vi "GetSystemDirectory.vi"() -> ()   [LabVIEW 2011]
doc: "Uses an API call to retrieve the path to thesystem directory."
uses:
  kernel32.dll
panel:
  out "error out":errorcluster
  in  "error in (no error)":errorcluster
  out "System Directory Path":string
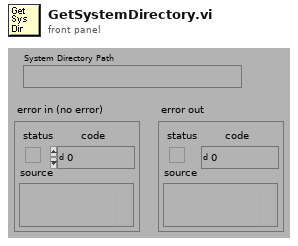
[diagram p1: front panel]
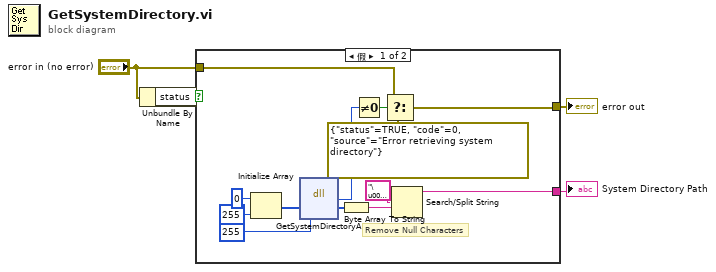
[diagram p0: block diagram]
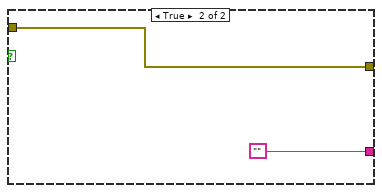
[diagram p2: hidden frame]
diagram:
  n1 = Unbundle By Name("error in (no error)") -> ("status"=w3:bool)
  n2 = case shown="假" w3 {
    tunnel: [w12 "" ("string")] -> w4
    tunnel: "error in (no error)" -> [w7 w19]
    tunnel: [w6 w19] -> w1
    frame False {
      # "Remove Null Characters"
      n3 = Initialize Array(u8 0, 255) -> (w15:u8[])
      n4 = dll-call lib="kernel32.dll" fn="GetSystemDirectoryA" label="Get System Directory"("lpBuffer"=w15, "nSize"=u32 255) -> (w9:u8, "lpBuffer"=w16:u8[])  [unwired: 4 in, 2 out]
      n5 = Byte Array To String(unsigned byte array=w16) -> (string=w14:string)
      n6 = Not Equal To 0?(x=w9) -> (x != 0?=w8:bool)
      n7 = Select(t=w7, s=w8, f=errorcluster {"status"=TRUE, "code"=0, "source"="Error retrieving system directory"}) -> (s? t:f=w6:errorcluster)
      n8 = Search/Split String(string=w14, search string/char (-)="\u0000" ("regular expression")) -> (substring before match=w12:string)  [unwired: 1 in, 2 out]
    }
    frame True {
    }
  }
  "System Directory Path" <- w4
  "error out" <- w1
